vi "OAT Full Spectrum (1 Pair Waveforms).vi"(0 "scaled signal X [EU]":waveform(dbl), 1 "scaled signal Y [EU]":waveform(dbl), 2 "window (Hanning)":T10=1 items=["None"=0, "Hanning"=1, "Hamming"=2, "Blackman-Harris"=3, "Exact Blackman"=4, "Blackman"=5, "Flat Top"=6, "4 Term B-Harris "=7, "7 Term B-Harris"=8, "Low Sidelobe"=9, "Force - Exponential"=10, "Blackman Nuttall"=11, "Triangle"=30, "Bartlett-Hanning"=31, "Bohman"=32, "Parzen"=33, "Welch"=34, "Kaiser"=60, "Dolph-Chebyshev"=61, "Gaussian"=62], 4 "view":T8={"dB On (F)"=FALSE, "unwrap phase (F)"=FALSE, "convert to degree (T)"=TRUE}, 5 "error in (no error)":errorcluster, 6 "rotation direction (CCW)":u16(ring) items=["CCW", "CW"], 7 "averaging parameters":T9={"averaging mode"=enum."No averaging", "weighting mode"=enum."Exponential", "number of averages"=10, "linear mode"=enum."One shot"}, 9 "restart averaging (F)":bool) -> (11 "averaging done":bool, 13 "averages completed":dbl, 14 "full spectrum":T7, 15 "magnitude unit label":string, 16 "phase lag":cluster{"f0":dbl, "df":dbl, "phase":dbl[]} {"phase" format="%.2f"; "df" format="%.2f"; "f0" format="%.2f"}, 17 "phase unit label":string, 18 "spectrum info":T1={"channel name"="", "description"="", "x-axis units"=0, "spectral info"={"spectrum type"=enum."Power [Magnitude^2]", "linear/dB"=enum."linear", "window"=0, "window size"=0, "FFT size"=0}, "engineering units"=0, "custom label"="", "dB reference [EU]"=0.0, "peak units"=enum."rms", "weighting filter"=0, "spectral density?"=FALSE, "unit label"="", "spectrum skewed?"=FALSE, "complimentary spectrum units"=enum."none"} {"x-axis units" items=["Time (s)"=0, "Frequency-CB (Hz)"=1, "Frequency-CPB (Hz)"=1248, "Frequency-Arbitrary (Hz)"=2357, "Quefrency (s)"=2, "Revolutions (rev)"=3, "Order"=4, "Speed (RPM)"=11, "Speed (rad/s)"=21, "Index"=65535]; "weighting filter" items=["Linear", "A-weighting", "B-weighting", "C-weighting", "ITU-R 468-4", "Dolby", "CCITT", "C-message", "Wb", "Wc", "Wd", "We", "Wf", "Wh", "Wj", "Wk", "Wm", "AES17 20 kHz lowpass", "AES17 40 kHz lowpass", "AES17 20 kHz highpass", "AES17 40 kHz highpass"]; "dB reference [EU]" format="%.2f"; "engineering units" items=["custom..."=0, "V"=1, "A"=21, "C"=30, "pC"=31, "s"=32, "-"=29, "Pa"=2, "N"=20, "g"=3, "m/s^2"=4, "m/s"=5, "m"=6, "mm/s"=12, "mm"=13, "micron/s"=14, "micron"=15, "in/s^2"=7, "in/s"=8, "in"=9, "mil/s"=10, "mil"=11, "rad/s^2"=16, "rad/s"=17, "rad"=18, "deg/s^2"=26, "deg/s"=27, "deg"=28, "RPM"=22, "cycle/s^2"=23, "Hz"=24, "cycle"=25, "strain"=19]; "spectral info"."window" items=["None "=0, "Hanning"=1, "Hamming"=2, "Blackman-Harris"=3, "Exact Blackman"=4, "Blackman"=5, "Flat Top"=6, "4 Term B-Harris "=7, "7 Term B-Harris"=8, "Low Sidelobe"=9, "Force - Exponential"=10, "Gaussian"=62]}, 19 "error out":errorcluster)   [LabVIEW 2017, in "SoundVib_OrderTracking.lvlib"]
doc: "This VI computes the full spectrum of a probe pair. The full spectrum provides information on the amplitude of vibration as well as the orbit eccentricity and direction of precession for each frequency/order component."
uses:
  <vilib>/addons/Sound and Vibration/Order Analysis/Resample Order Tracking/SoundVib_OrderTracking.lvlib
  <vilib>/addons/_NISVFA/_Shared subVIs/Controls/svc_Window [Dual FFT].ctl
  <vilib>/addons/_NISVFA/_Shared subVIs/Controls/svc_Spectrum Info.ctl
  <vilib>/addons/_NISVFA/_Shared subVIs/Controls/svc_X-Axis Units.ctl
  <vilib>/addons/_NISVFA/_Shared subVIs/Controls/svc_Spectrum Type.ctl
  <vilib>/addons/_NISVFA/_Shared subVIs/Controls/svc_Engineering Units Text Ring.ctl
  <vilib>/addons/_NISVFA/_Shared subVIs/Controls/svc_Weighting Filter Text Ring.ctl
  <vilib>/addons/_NISVFA/_Shared subVIs/Controls/svc_Complimentary Spectrum Units.ctl
  <vilib>/addons/_NISVFA/_Spectrum Processing/SVFA Unit Conversion (1 Ch).vi
  <vilib>/addons/_NISVFA/_Shared subVIs/Common/svc_Spectrum Units.vi
  <vilib>/addons/_NISVFA/_Spectrum Processing/subVIs/svfa_Conversion Utility (spectrum info).vi
  <vilib>/addons/_NISVFA/_Spectrum Processing/subVIs/svfa_Peak to RMS to Peak2Peak.vi
  <vilib>/addons/_NISVFA/_Spectrum Processing/subVIs/svfa_Mag to Mag2.vi
  <vilib>/addons/_NISVFA/_Spectrum Processing/subVIs/svfa_Linear to dB.vi
  <vilib>/addons/_NISVFA/_Spectrum Processing/subVIs/svfa_dBrefA to dBrefB.vi
  <vilib>/addons/_NISVFA/_Spectrum Processing/subVIs/svfa_Spectrum to Spectral Density.vi
  <vilib>/addons/_NISVFA/_Shared subVIs/Common/svc_Get Weighting Enum and Labels.vi
  <vilib>/addons/_NISVFA/_Shared subVIs/Common/svc_Unit Label Lexical Class.vi
  <vilib>/addons/_NISVFA/_Shared subVIs/Common/svc_Engineering Units to Unit Label.vi
  <vilib>/addons/_NISVFA/_Shared subVIs/Common/svc_Format Value (DBL).vi
  <vilib>/addons/_NISVFA/_Shared subVIs/Common/svc_Window Parameters.vi
  <vilib>/addons/_NISVFA/_Spectrum Processing/SVFA Wrap or Unwrap Phase (1 Ch).vi
  <vilib>/addons/_NISVFA/_Spectrum Processing/SVFA Phase Unit Conversion (1 Ch).vi
  <vilib>/addons/_NISVFA/_Spectrum Processing/SVFA Unit Conversion (Complex) (1 Ch).vi
  <vilib>/addons/_NISVFA/_Baseband FFT/SVFA FFT Spectrum (Complex) (1 Ch).vi
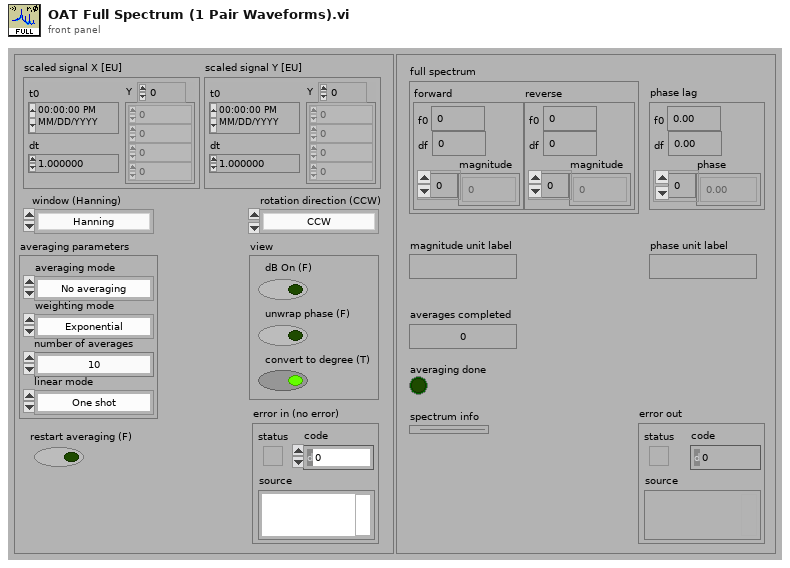
[diagram p1: front panel]
types:
  T1 = typedef "svc_Spectrum Info.ctl" = cluster{"channel name":string, "description":string, "x-axis units":T2, "spectral info":cluster{"spectrum type":T3, "linear/dB":enum16{"linear", "dB"}, "window":u16, "window size":i32, "FFT size":i32}, "engineering units":T4, "custom label":string, "dB reference [EU]":dbl, "peak units":enum16{"rms", "peak", "peak-peak"}, "weighting filter":T5, "spectral density?":bool, "unit label":string, "spectrum skewed?":bool, "complimentary spectrum units":T6}
  T2 = typedef "svc_X-Axis Units.ctl" = u16
  T3 = typedef "svc_Spectrum Type.ctl" = enum16{"FFT Spectrum [complex]", "Amplitude [Magnitude]", "Power [Magnitude^2]", "Cross Spectrum [complex]", "Frequency Response [Complex]"}
  T4 = typedef "svc_Engineering Units Text Ring.ctl" = u16
  T5 = typedef "svc_Weighting Filter Text Ring.ctl" = u16
  T6 = typedef "svc_Complimentary Spectrum Units.ctl" = enum16{"none", "radians", "degrees", "cycles", "imaginary"}
  T7 = cluster{"forward":cluster{"f0":dbl, "df":dbl, "magnitude":dbl[]}, "reverse":cluster{"f0":dbl, "df":dbl, "magnitude":dbl[]}}
  T8 = cluster{"dB On (F)":bool, "unwrap phase (F)":bool, "convert to degree (T)":bool}
  T9 = cluster{"averaging mode":enum16{"No averaging", "Vector averaging", "RMS averaging", "Peak hold"}, "weighting mode":enum16{"Linear", "Exponential"}, "number of averages":u32, "linear mode":enum16{"One shot", "Auto restart"}}
  T10 = typedef "svc_Window [Dual FFT].ctl" = u32
  T11 = cluster{"linear/dB":enum16{"no change", "linear", "dB"}, "dB reference (0: no change)":dbl, "power/magnitude":enum16{"no change", "power", "magnitude"}, "view":enum16{"no change", "rms", "peak", "peak-peak"}}
  T12 = enum16{"No change", "Radians", "Degrees", "Cycles"}
  T13 = enum16{"No change", "Unwrap", "Wrap: -360 to 0", "Wrap: -270 to 90", "Wrap: -180 to 180", "Wrap: -90 to 270", "Wrap: 0 to 360", "Wrap: custom range"}
  T14 = cluster{"dB On (T)":bool, "unwrap phase (F)":bool, "convert to degree (T)":bool}
  T15 = cluster{"forward":cluster{"x0":dbl, "dx":dbl, "magnitude":dbl[]}, "reverse":cluster{"x0":dbl, "dx":dbl, "magnitude":dbl[]}}
  T16 = cluster{"complex spectrum response":cluster{"f0":dbl, "df":dbl, "complex spectrum":cdb[]}, "spectrum info":T1}
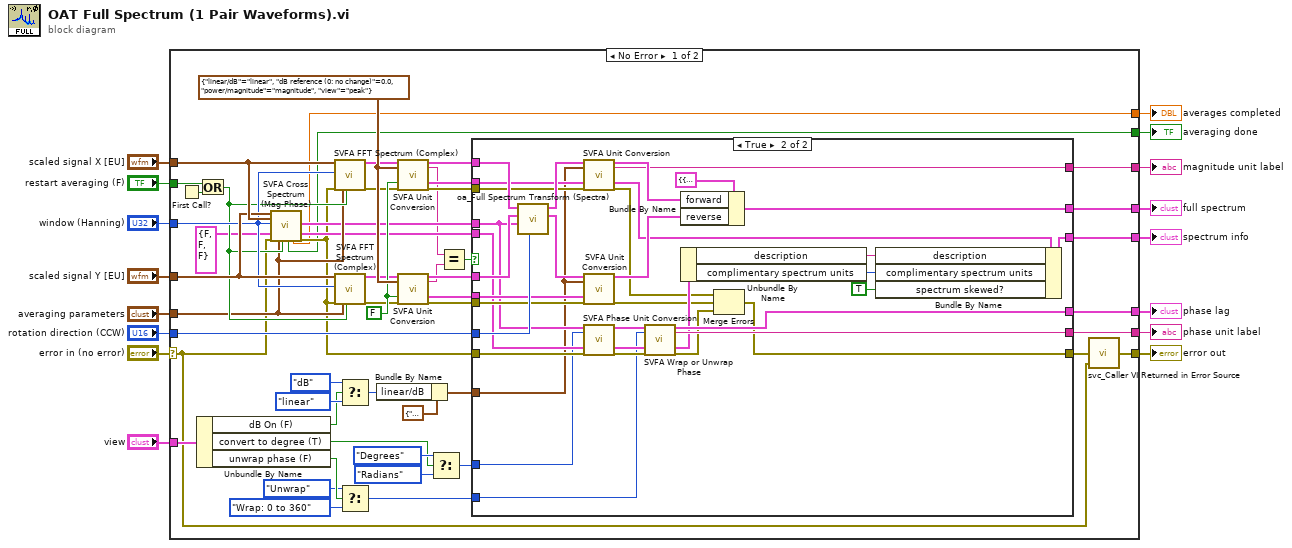
[diagram p0: block diagram]
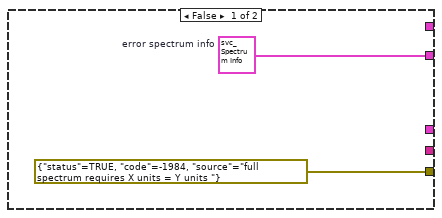
[diagram p2: hidden frame]
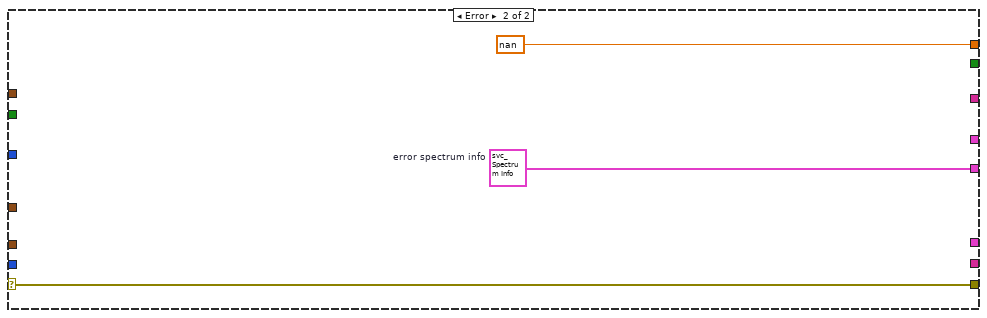
[diagram p3: hidden frame]
diagram:
  n1 = case shown="No Error" "error in (no error)" {
    selector: "error in (no error)" -> [w17 w108]
    tunnel: "window (Hanning)" -> [w66 _]
    tunnel: "averaging parameters" -> [w53 _]
    tunnel: "view" -> [w43 _]
    tunnel: [w18 w108] -> w13
    tunnel: [w24 _] -> w12
    tunnel: [w26 _] -> w11
    tunnel: "scaled signal X [EU]" -> [w68 _]
    tunnel: "scaled signal Y [EU]" -> [w67 _]
    tunnel: [w47 _] -> w7
    tunnel: [w25 _] -> w6
    tunnel: [w28 nan ("averages completed")] -> w5
    tunnel: [w27 _] -> w4
    tunnel: [w23 w106] -> w3
    tunnel: "restart averaging (F)" -> [w64 _]
    tunnel: "rotation direction (CCW)" -> [w54 _]
    frame No Error {
      w60 = T11 {"linear/dB"=enum."linear", "dB reference (0: no change)"=0.0, "power/magnitude"=enum."magnitude", "view"=enum."peak"} ("desired scaling")
      w59 = FALSE ("convert to degree (T)")
      n2 = First Call?() -> (First Call?: T/F=w65:bool)
      n3 = Unbundle By Name(w43) -> ("dB On (F)"=w31:bool, "convert to degree (T)"=w35:bool, "unwrap phase (F)"=w42:bool)
      n4 = Or(x=w64, y=w65) -> (x .or. y?=w63:bool)
      n5 = call <vilib>:"SVFA Cross Spectrum (Mag-Phase).vi"("scaled signal X [EUx]"=w67, "scaled signal Y [EUy]"=w68, "window"=w66, "view"=T14 {"dB On (T)"=FALSE, "unwrap phase (F)"=FALSE, "convert to degree (T)"=FALSE}, "error in (no error)"=w17, "averaging parameters"=w53, "restart averaging (F)"=w63) -> ("averaging done"=w27:bool, "averages completed"=w28:dbl, "phase [degrees]"=w46:cluster{"f0":dbl, "df":dbl, "phase":dbl[]}, "spectrum info"=w45:T1, "error out"=w44:errorcluster)  [unwired: 5 in, 3 out]
      n6 = call-poly <vilib>:"SVFA FFT Spectrum (Complex).vi"("scaled signal [EU]"=w68, "window"=w66, "error in"=w44, "averaging parameters"=w53, "restart averaging (F)"=w63) -> ("complex spectrum"=w57:T16, "error out"=w56:errorcluster)  [unwired: 11 in, 2 out]
      n7 = call-poly <vilib>:"SVFA FFT Spectrum (Complex).vi"("scaled signal [EU]"=w67, "window"=w66, "error in"=w44, "averaging parameters"=w53, "restart averaging (F)"=w63) -> ("complex spectrum"=w58:T16, "error out"=w55:errorcluster)  [unwired: 11 in, 2 out]
      n8 = Select(t=enum16{"no change", "linear", "dB"}."dB" ("linear/dB"), s=w31, f=enum16{"no change", "linear", "dB"}."linear" ("linear/dB")) -> (s? t:f=w30:enum16{"no change", "linear", "dB"})
      n9 = Select(t=T13."Unwrap" ("desired wrapping"), s=w42, f=T13."Wrap: 0 to 360" ("desired wrapping")) -> (s? t:f=w39:T13)
      n10 = Bundle By Name(cluster=T11 {"linear/dB"=enum."no change", "dB reference (0: no change)"=0.0, "power/magnitude"=enum."no change", "view"=enum."no change"} ("desired scaling"), "linear/dB"=w30) -> (w29:T11)
      n11 = call-poly <vilib>:"SVFA Unit Conversion.vi"("complex spectrum"=w57, "desired scaling"=w60, "convert to degree (T)"=w59, "error in (no error)"=w56) -> ("converted spectrum"=w52:cluster{"x0":dbl, "dx":dbl, "magnitude":dbl[]}, "magnitude unit label"=w22:string, "spectrum info out"=w50:T1, "error out"=w48:errorcluster)  [unwired: 10 in, 2 out]
      n12 = call-poly <vilib>:"SVFA Unit Conversion.vi"("complex spectrum"=w58, "desired scaling"=w60, "convert to degree (T)"=w59, "error in (no error)"=w55) -> ("converted spectrum"=w61:cluster{"x0":dbl, "dx":dbl, "magnitude":dbl[]}, "magnitude unit label"=w21:string, "spectrum info out"=w51:T1, "error out"=w49:errorcluster)  [unwired: 10 in, 2 out]
      n13 = Select(t=T12."Degrees" ("desired units"), s=w35, f=T12."Radians" ("desired units")) -> (s? t:f=w36:T12)
      n14 = Equal?(x=w22, y=w21) -> (x = y?=w20:bool)
      n15 = case shown="True" w20 {
        tunnel: [errorcluster {"status"=TRUE, "code"=-1984, "source"="full spectrum requires X units = Y units "} ("error out") w71] -> w19
        tunnel: w61 -> [_ w104]
        tunnel: w54 -> [_ w103]
        tunnel: w52 -> [_ w102]
        tunnel: w51 -> [_ w99]
        tunnel: w50 -> [_ w98]
        tunnel: w49 -> [_ w97]
        tunnel: w48 -> [_ w96]
        tunnel: [_ w93] -> w47
        tunnel: w46 -> [_ w92]
        tunnel: w45 -> [_ w91]
        tunnel: w44 -> [_ w87]
        tunnel: w39 -> [_ w86]
        tunnel: w36 -> [_ w85]
        tunnel: w29 -> [_ w84]
        tunnel: [_ w83] -> w26
        tunnel: [_ w82] -> w25
        tunnel: [_ w81] -> w24
        tunnel: [w69 w75] -> w23
        frame False {
          w69 = T1 {"channel name"="Error", "description"="Error", "x-axis units"=99, "spectral info"={"spectrum type"=enum."Power [Magnitude^2]", "linear/dB"=enum."linear", "window"=99, "window size"=-1, "FFT size"=-1}, "engineering units"=0, "custom label"="Error", "dB reference [EU]"=0.0, "peak units"=enum."rms", "weighting filter"=0, "spectral density?"=FALSE, "unit label"="Error", "spectrum skewed?"=FALSE, "complimentary spectrum units"=enum."none"}  # error spectrum info
        }
        frame True {
          n16 = call <vilib>:"oa_Full Spectrum Transform (Spectra).vi"("direction"=w103, "phase lag spectrum (X-Y)"=w92, "Y magnitude spectrum"=w104, "X magnitude spectrum"=w102) -> ("reverse precession spectrum"=w100:cluster{"x0":dbl, "dx":dbl, "magnitude":dbl[]}, "forward precession spectrum"=w101:cluster{"x0":dbl, "dx":dbl, "magnitude":dbl[]})  [unwired: 6 in]
          n17 = call-poly <vilib>:"SVFA Unit Conversion.vi"("spectrum"=w101, "desired scaling"=w84, "spectrum info in"=w98, "error in (no error)"=w96) -> ("converted spectrum"=w95:cluster{"x0":dbl, "dx":dbl, "magnitude":dbl[]}, "unit label"=w93:string, "spectrum info out"=w76:T1, "error out"=w74:errorcluster)  [unwired: 12 in]
          n18 = call-poly <vilib>:"SVFA Unit Conversion.vi"("spectrum"=w100, "desired scaling"=w84, "spectrum info in"=w99, "error in (no error)"=w97) -> ("converted spectrum"=w94:cluster{"x0":dbl, "dx":dbl, "magnitude":dbl[]}, "error out"=w73:errorcluster)  [unwired: 12 in, 2 out]
          n19 = call-poly <vilib>:"SVFA Phase Unit Conversion.vi"("phase spectrum"=w92, "desired units"=w85, "spectrum info in"=w91, "error in (no error)"=w87) -> ("converted phase spectrum"=w90:cluster{"f0":dbl, "df":dbl, "phase":dbl[]}, "spectrum info out"=w89:T1, "error out"=w88:errorcluster)  [unwired: 12 in, 1 out]
          n20 = call-poly <vilib>:"SVFA Wrap or Unwrap Phase.vi"("phase spectrum in"=w90, "desired wrapping"=w86, "spectrum info"=w89, "error in (no error)"=w88) -> ("phase spectrum out"=w81:cluster{"f0":dbl, "df":dbl, "phase":dbl[]}, "unit label"=w82:string, "dup spectrum info"=w80:T1, "error out"=w72:errorcluster)  [unwired: 12 in]
          n21 = Bundle By Name(cluster=T15 {"forward"={"x0"=0.0, "dx"=0.0, "magnitude"=[]}, "reverse"={"x0"=0.0, "dx"=0.0, "magnitude"=[]}}, "forward"=w95, "reverse"=w94) -> (w83:T15)
          n22 = Unbundle By Name(w80) -> ("description"=w79:string, "complimentary spectrum units"=w78:T6)
          n23 = Merge Errors(w74, w73, w72) -> (w71:errorcluster)
          n24 = Bundle By Name(cluster=w76, "description"=w79, "complimentary spectrum units"=w78, "spectrum skewed?"=TRUE) -> (w75:T1)
        }
      }
      n25 = call <vilib>:"svc_Caller VI Returned in Error Source.vi"("warning input to caller"=w17, "error in (no error)"=w19) -> ("error out"=w18:errorcluster)  [unwired: 3 in]
    }
    frame Error {
      w106 = T1 {"channel name"="Error", "description"="Error", "x-axis units"=99, "spectral info"={"spectrum type"=enum."Power [Magnitude^2]", "linear/dB"=enum."linear", "window"=99, "window size"=-1, "FFT size"=-1}, "engineering units"=0, "custom label"="Error", "dB reference [EU]"=0.0, "peak units"=enum."rms", "weighting filter"=0, "spectral density?"=FALSE, "unit label"="Error", "spectrum skewed?"=FALSE, "complimentary spectrum units"=enum."none"}  # error spectrum info
    }
  }
  "error out" <- w13
  "phase lag" <- w12
  "full spectrum" <- w11
  "magnitude unit label" <- w7
  "phase unit label" <- w6
  "averages completed" <- w5
  "averaging done" <- w4
  "spectrum info" <- w3
